vi "CMD_Loop.vi"() -> ()   [LabVIEW 2020, in "MotionMaster_SubCMD.lvlib"]
uses:
  MotionMaster_SubCMD.lvlib
  Cluster_CMD_CMD_Data.ctl
  ENUM_CMD_Mode.ctl
  ENUM_Pose List.ctl
  Shared Code/TypeDefs/Cluster_Pose Positions.ctl
  Shared Code/TypeDefs/Cluster_MotionMaster_Config Data.ctl
  Shared Code/TypeDefs/Cluster_Pose Name and  Data.ctl
  Lift/Cluster_CMD_ACT_Data.ctl
  Shared Code/TypeDefs/ENUM_Lift_CMD_Mode Select.ctl
  Wrist/Cluster_CMD_ACT_Data.ctl
  Shared Code/TypeDefs/ENUM_Wrist_CMD_Mode Select.ctl
  Extention/Cluster_CMD_ACT_Data.ctl
  Shared Code/TypeDefs/ENUM_Extend_CMD_Mode Select.ctl
  Shared Code/TypeDefs/Cluster_MotionMaster Output.ctl
  ENUM_CMD_State.ctl
  Shared Code/TypeDefs/Cluster_Lift_HW Outputs.ctl
  Shared Code/TypeDefs/Cluster_FX Sensor Values.ctl
  Shared Code/TypeDefs/Cluster_FX CloseLoop Values.ctl
  Shared Code/TypeDefs/Cluster_FX Limit Switchs.ctl
  Shared Code/TypeDefs/Cluster_FX Current Values.ctl
  Shared Code/TypeDefs/Cluster_FX Integrated Sensor Values.ctl
  Shared Code/TypeDefs/Cluster_Lift_SW Output Data.ctl
  Shared Code/TypeDefs/Cluster_Wrist HW Outputs.ctl
  Shared Code/TypeDefs/Cluster_Wrist_SW Output Data.ctl
  Shared Code/TypeDefs/Cluster_Extend HW Outputs.ctl
  Shared Code/TypeDefs/Cluster_Extend_SW Output Data.ctl
  ENUM_CMD_Action.ctl
  f0e3bde4-301b-4f9a-9fe5-06516af7aa09.vi
  30192d10-bba2-489c-a06e-f8bf0f82b926.vi
  77e6cb1f-e30f-4d03-9d33-3a90b036f1c5.vi
  37f9d8cc-f1a8-4678-af2d-79a500a222a4.vi
  5685669b-8200-4586-8aad-fb6ccbc2f0c7.vi
  9608b361-7489-41d5-b543-0e30ed415d4d.vi
  543e74ff-1c65-4f6d-a6cc-884adac36b74.vi
  2e6b047f-cb73-4edf-a9eb-2cc3cf528fa5.vi
  543e74ff-1c65-4f6d-a6cc-884adac36b74.vi/f38ca901-adc1-4ad8-996e-31aeb746ae36.vi
  543e74ff-1c65-4f6d-a6cc-884adac36b74.vi/958b2683-dd4b-41b7-8ed1-41c95f63cef0.vi
  2e6b047f-cb73-4edf-a9eb-2cc3cf528fa5.vi/f38ca901-adc1-4ad8-996e-31aeb746ae36.vi
  2e6b047f-cb73-4edf-a9eb-2cc3cf528fa5.vi/958b2683-dd4b-41b7-8ed1-41c95f63cef0.vi
  543e74ff-1c65-4f6d-a6cc-884adac36b74.vi/f38ca901-adc1-4ad8-996e-31aeb746ae36.vi/1c6bd52c-bbca-4d4a-a290-93ea2703fded.vi
  543e74ff-1c65-4f6d-a6cc-884adac36b74.vi/f38ca901-adc1-4ad8-996e-31aeb746ae36.vi/47c2b0d5-b5fa-444e-9535-611565d375db.vi
  2e6b047f-cb73-4edf-a9eb-2cc3cf528fa5.vi/f38ca901-adc1-4ad8-996e-31aeb746ae36.vi/1c6bd52c-bbca-4d4a-a290-93ea2703fded.vi
  2e6b047f-cb73-4edf-a9eb-2cc3cf528fa5.vi/f38ca901-adc1-4ad8-996e-31aeb746ae36.vi/47c2b0d5-b5fa-444e-9535-611565d375db.vi
  Global_CMD_CMD_Data In.vi
  Utility/Global_STOP.vi
  Lift/Global_ACT_Data Out.vi
  Wrist/Global_ACT_Data Out.vi
  Extention/Global_ACT_Data Out.vi
  <vilib>/Utility/Data Type/Get Type Information.vi
  <vilib>/Utility/error.llb/Trim Whitespace.vi
  Shared Code/Utility/RWA/RWA/File/RWA_PC FIle Read String.vi
  Shared Code/Utility/RWA/RWA/Read Write Anything/RWA_File String.vi
  Shared Code/Utility/RWA/RWA/File/RWA_PC File Write String.vi
  Global_CMD_Data Out.vi
  Lift/Global_CMD_ACT_Data In.vi
  Extention/Global_CMD_ACT_Data In.vi
  Wrist/Global_CMD_ACT_Data In.vi
  <vilib>/Comparison/Equal/Equal Functor/Equal Functor.lvclass
  Extention/Extend_ACT.lvlib
  Wrist/Wrist_ACT.lvlib
  Lift/Lift_ACT.lvlib
panel:
  out "Message":string
  out "Pose Index":i32
  out "Pose Targets":T1[](array[typedef])
  in  "Read Saved Config":bool
  in  "Update Config":bool
  out "MotionMaster_Output":T2
  out "Extend Position":i32
  out "Wrist @Positon":bool
  out "Wrist Position":i32
  out "Extend @ Positon":bool
  out "Lift Position":i32
  out "Lift @ Positon":bool
  out "Extend CMD":T4
  out "Wrist CMD":T6
  out "Lift CMD":T8
  out "CMD.ENABLE":bool
  out "Current Time":timestamp
  in  "Config Data":T10
  out "CMD":T12
  out "Cycle Time (S)":dbl format="%.3g"
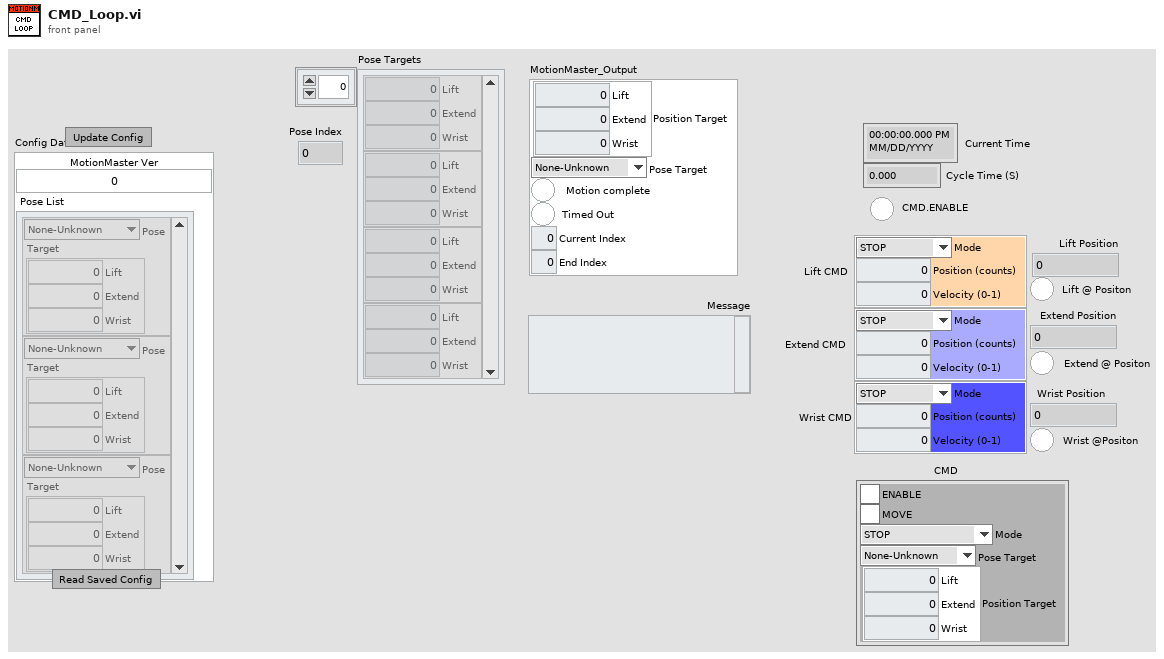
[diagram p1: front panel]
types:
  T1 = typedef "Cluster_Pose Positions.ctl" = cluster{"Lift":i32, "Extend":i32, "Wrist":i32}
  T2 = typedef "Cluster_MotionMaster Output.ctl" = cluster{"Position Target":T1, "Pose Target":T3, "Motion complete":bool, "Timed Out":bool, "Current Index":i32, "End Index":i32}
  T3 = typedef "MotionMaster_SubCMD.lvlib/ENUM_Pose List.ctl" = enum16{"None-Unknown", "Intake", "Score High", "Score Mid", "Safe Position", "Home Pos"}
  T4 = typedef "Extend_ACT.lvlib/Cluster_CMD_ACT_Data.ctl" = cluster{"Mode":T5, "Position (counts)":i32, "Velocity (0-1)":dbl}
  T5 = typedef "ENUM_Extend_CMD_Mode Select.ctl" = enum16{"STOP", "Position", "Velocity", "Force Home"}
  T6 = typedef "Wrist_ACT.lvlib/Cluster_CMD_ACT_Data.ctl" = cluster{"Mode":T7, "Position (counts)":i32, "Velocity (0-1)":dbl}
  T7 = typedef "ENUM_Wrist_CMD_Mode Select.ctl" = enum16{"STOP", "Position", "Speed"}
  T8 = typedef "Lift_ACT.lvlib/Cluster_CMD_ACT_Data.ctl" = cluster{"Mode":T9, "Position (counts)":i32, "Velocity (0-1)":dbl}
  T9 = typedef "ENUM_Lift_CMD_Mode Select.ctl" = enum16{"STOP", "Position", "Percent out"}
  T10 = typedef "Cluster_MotionMaster_Config Data.ctl" = cluster{"MotionMaster Ver":u64, "Pose List":T11[]}
  T11 = typedef "Cluster_Pose Name and  Data.ctl" = cluster{"Pose":T3, "Target":T1}
  T12 = typedef "MotionMaster_SubCMD.lvlib/Cluster_CMD_CMD_Data.ctl" = cluster{"ENABLE":bool, "MOVE":bool, "Mode":T13, "Pose Target":T3, "Position Target":T1}
  T13 = typedef "MotionMaster_SubCMD.lvlib/ENUM_CMD_Mode.ctl" = enum16{"STOP", "Pose Target", "Position Target"}
  T14 = typedef "Cluster_Extend_SW Output Data.ctl" = cluster{"Enabled":bool, "Closed Loop":bool, "exAt Positon":bool}
  T15 = typedef "Cluster_Extend HW Outputs.ctl" = cluster{"CLosed Loop":T16, "Limit Switches":T17, "Current":T18, "FX Encoder":T19, "Cancoder":T20}
  T16 = typedef "Cluster_FX CloseLoop Values.ctl" = cluster{"Target":dbl, "Error":i32, "Error D":dbl, "I Accum":dbl}
  T17 = typedef "Cluster_FX Limit Switchs.ctl" = cluster{"FWD Closed":bool, "REV Closed":bool}
  T18 = typedef "Cluster_FX Current Values.ctl" = cluster{"Supply":dbl, "Stator":dbl}
  T19 = typedef "Cluster_FX Sensor Values.ctl" = cluster{"Position":i32, "Velocity":i32}
  T20 = typedef "Cluster_FX Integrated Sensor Values.ctl" = cluster{"Position":dbl, "Velocity":dbl, "Absolute":dbl}
  T21 = typedef "Cluster_Wrist_SW Output Data.ctl" = cluster{"Enabled":bool, "Closed Loop":bool, "Wr At Positon":bool}
  T22 = typedef "Cluster_Wrist HW Outputs.ctl" = cluster{"Encoder":T19, "CLosed Loop":T16, "Limit Switches":T17, "Current":T18, "Cancoder":T20}
  T23 = typedef "Cluster_Lift_SW Output Data.ctl" = cluster{"Enabled":bool, "Closed Loop":bool, "At Positon":bool}
  T24 = typedef "Cluster_Lift_HW Outputs.ctl" = cluster{"Encoder":T19, "CLosed Loop":T16, "Limit Switches":T17, "Current":T18, "Cancoder":T20}
  T25 = typedef "MotionMaster_SubCMD.lvlib/ENUM_CMD_State.ctl" = enum16{"Startup", "Configuring", "Waining For Enable", "Waiting For Start", "Setting Pose", "Moving to Pose", "Shutdown", "Completing Pose"}
  T26 = cluster{"State":T25, "Previous State":T25, "Current Time":timestamp, "Previous Time":timestamp, "Start Time":timestamp, "Target Time (ms)":u32, "Cycle Time(S)":dbl, "CMD":T12, "Lift CMD":T8, "Extend CMD":T4, "Wrist CMD":T6, "Previous CMD":T12, "Lift HW":T24, "Lift SW":T23, "Wrist HW":T22, "Wrist SW":T21, "Extend HW":T15, "Extend SW":T14, "Config Data":T10, "ALL At Positon":bool, "Pose Index":i32, "Update Display":bool, "MotionMaster_Output":T2, "Team Files Folder":path, "Pose Array":T1[], "PoseName":T3, "Current Pose":T1, "Valid Pose Target":bool, "Pose Wait Time":dbl, "Message":string, "Max Move Time":dbl}
  T27 = enum16{"Done", "First Call", "First Check", "Enabled"}
  T28 = enum16{"Done", "First Call", "First Check", "Enabled", "Move Enabled", "Positions Not Set"}
  T29 = enum16{"Done", "First Call", "First Check", "Enabled", "Move Enabled", "Positions Set", "Not At Positon"}
  T30 = typedef "MotionMaster_SubCMD.lvlib/ENUM_CMD_Action.ctl" = enum16{"No Action", "Reset Time", "Reset All", "Set Pose", "Config Pose Read File", "Build Pose List", "Config SW File Read", "Config SW File Save", "Config From FP"}
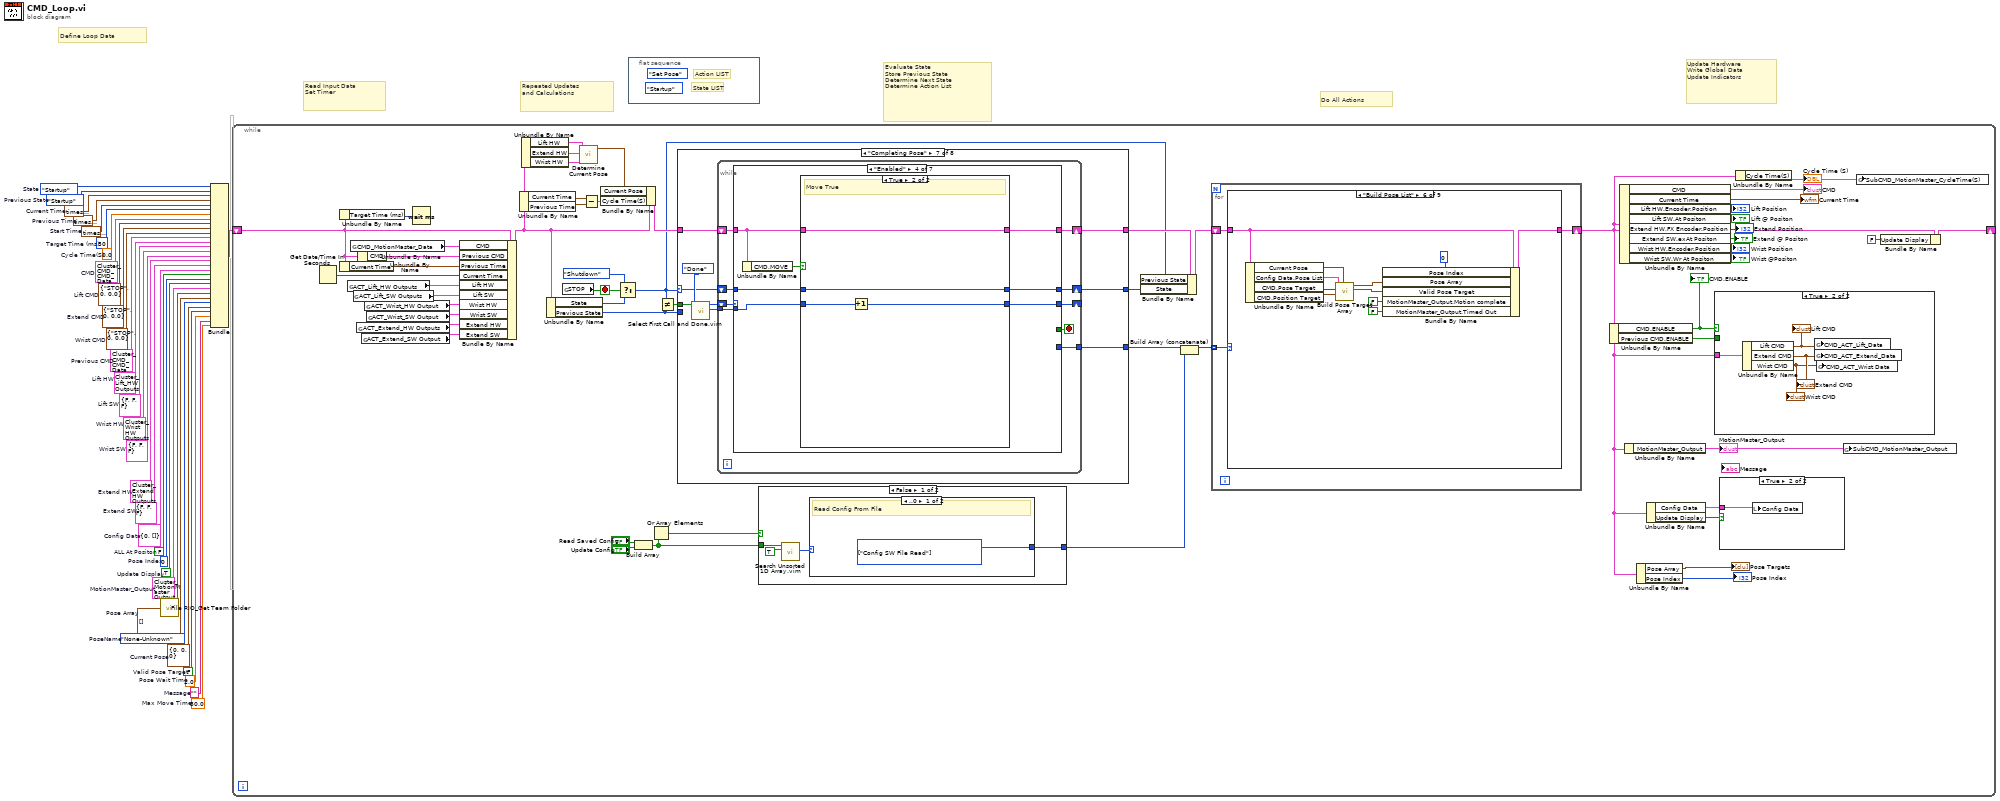
[diagram p0: block diagram]
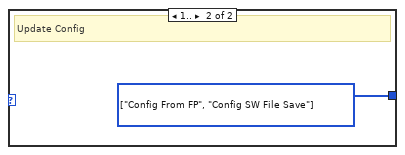
[diagram p2: hidden frame]
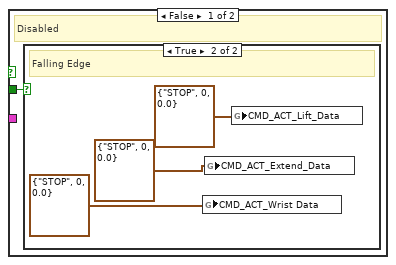
[diagram p5: hidden frame]
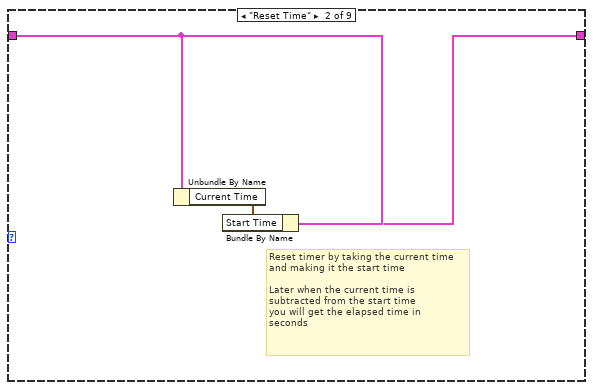
[diagram p8: hidden frame]
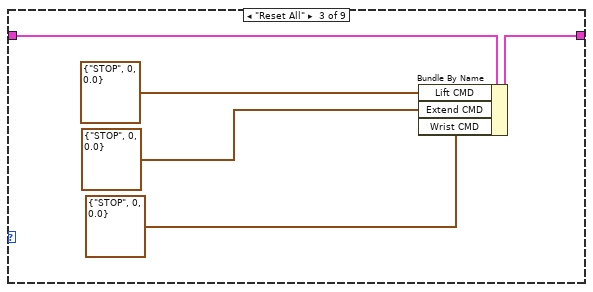
[diagram p9: hidden frame]
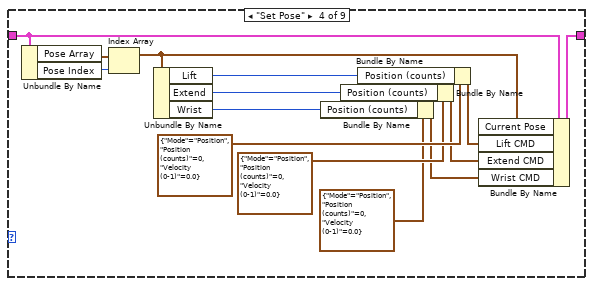
[diagram p10: hidden frame]
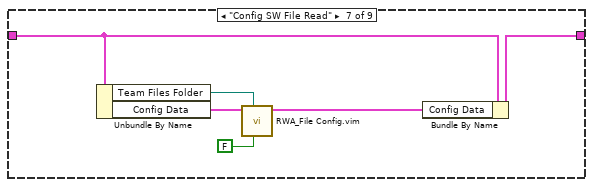
[diagram p12: hidden frame]
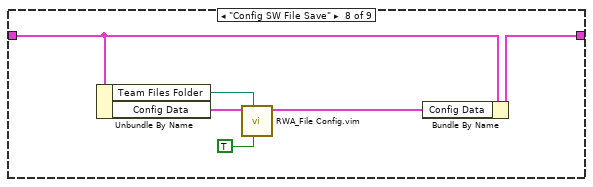
[diagram p13: hidden frame]
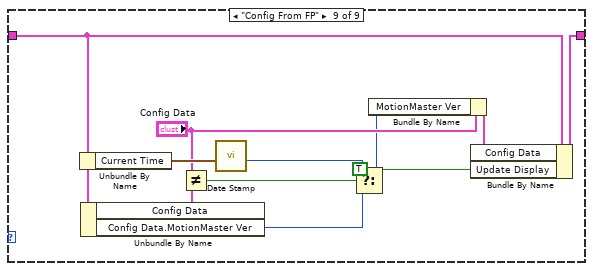
[diagram p14: hidden frame]
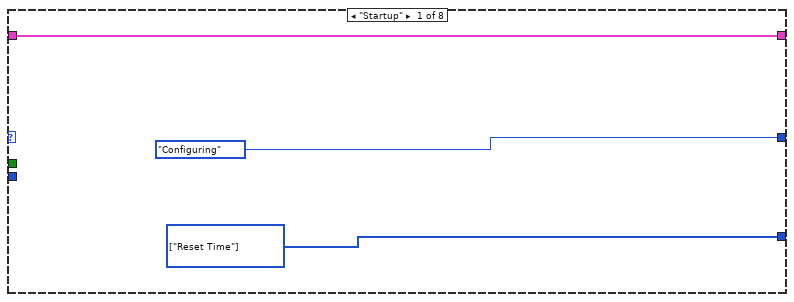
[diagram p15: hidden frame]
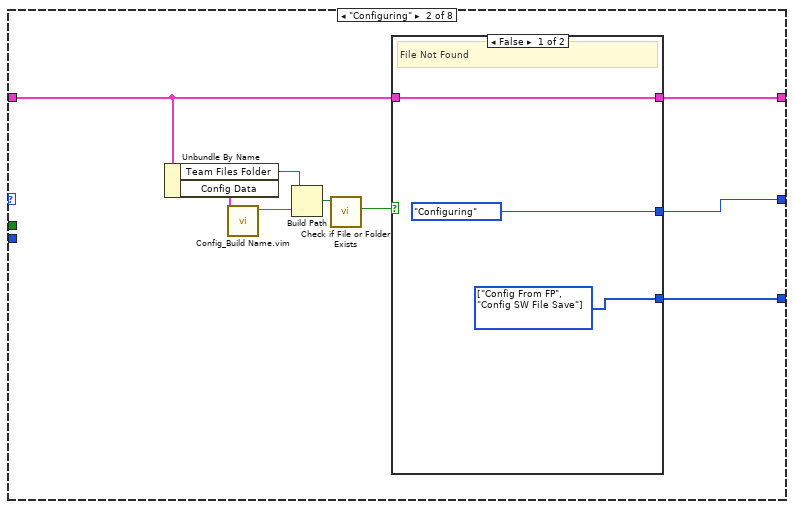
[diagram p16: hidden frame]
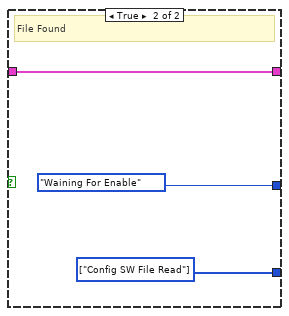
[diagram p17: hidden frame]
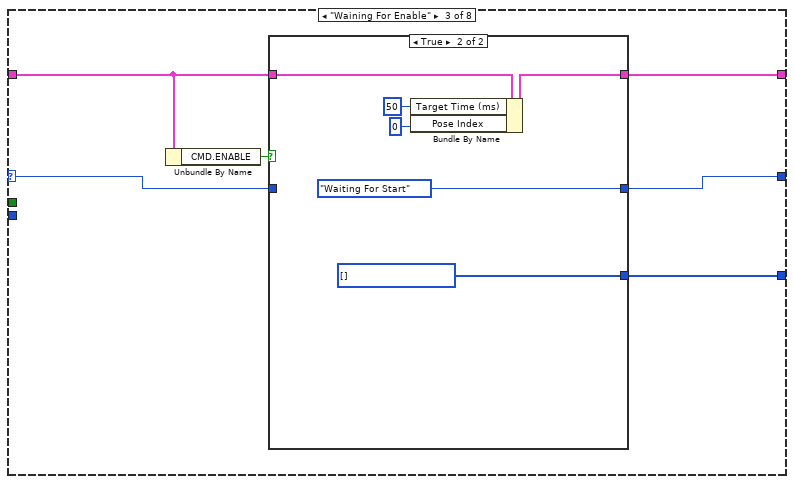
[diagram p18: hidden frame]
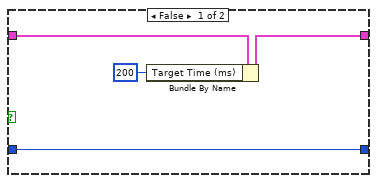
[diagram p19: hidden frame]
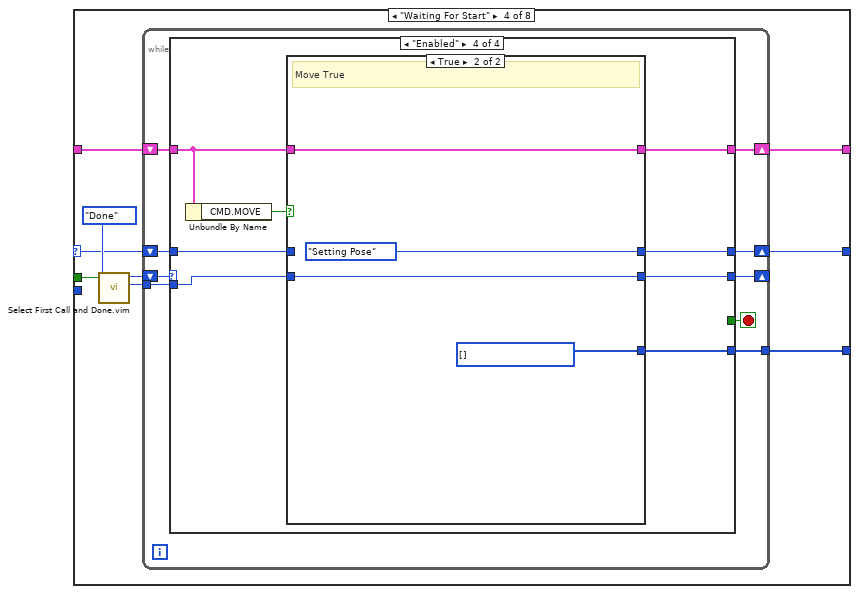
[diagram p20: hidden frame]
diagram:
  w1 = 30.0  # Max Move Time
  w2 = ""  # Message
  w3 = 2.0  # Pose Wait Time
  w4 = FALSE  # Valid Pose Target
  w5 = T1 {"Lift"=0, "Extend"=0, "Wrist"=0}  # Current Pose
  w6 = ENUM_Pose_List."None-Unknown"  # PoseName
  w8 = T1[] []  # Pose Array
  w10 = T2 {"Position Target"={"Lift"=0, "Extend"=0, "Wrist"=0}, "Pose Target"=enum."None-Unknown", "Motion complete"=FALSE, "Timed Out"=FALSE, "Current Index"=0, "End Index"=0}  # MotionMaster_Output
  w11 = TRUE  # Update Display
  w7 = 0  # Pose Index
  w12 = FALSE  # ALL At Positon
  w13 = T10 {"MotionMaster Ver"=0, "Pose List"=[]}  # Config Data
  w14 = T14 {"Enabled"=FALSE, "Closed Loop"=FALSE, "exAt Positon"=FALSE}  # Extend SW
  w15 = T15 {"CLosed Loop"={"Target"=0.0, "Error"=0, "Error D"=0.0, "I Accum"=0.0}, "Limit Switches"={"FWD Closed"=FALSE, "REV Closed"=FALSE}, "Current"={"Supply"=0.0, "Stator"=0.0}, "FX Encoder"={"Position"=0, "Velocity"=0}, "Cancoder"={"Position"=0.0, "Velocity"=0.0, "Absolute"=0.0}}  # Extend HW
  w16 = T21 {"Enabled"=FALSE, "Closed Loop"=FALSE, "Wr At Positon"=FALSE}  # Wrist SW
  w17 = T22 {"Encoder"={"Position"=0, "Velocity"=0}, "CLosed Loop"={"Target"=0.0, "Error"=0, "Error D"=0.0, "I Accum"=0.0}, "Limit Switches"={"FWD Closed"=FALSE, "REV Closed"=FALSE}, "Current"={"Supply"=0.0, "Stator"=0.0}, "Cancoder"={"Position"=0.0, "Velocity"=0.0, "Absolute"=0.0}}  # Wrist HW
  w18 = T23 {"Enabled"=FALSE, "Closed Loop"=FALSE, "At Positon"=FALSE}  # Lift SW
  w19 = T24 {"Encoder"={"Position"=0, "Velocity"=0}, "CLosed Loop"={"Target"=0.0, "Error"=0, "Error D"=0.0, "I Accum"=0.0}, "Limit Switches"={"FWD Closed"=FALSE, "REV Closed"=FALSE}, "Current"={"Supply"=0.0, "Stator"=0.0}, "Cancoder"={"Position"=0.0, "Velocity"=0.0, "Absolute"=0.0}}  # Lift HW
  w20 = T12 {"ENABLE"=FALSE, "MOVE"=FALSE, "Mode"=enum."STOP", "Pose Target"=enum."None-Unknown", "Position Target"={"Lift"=0, "Extend"=0, "Wrist"=0}}  # Previous CMD
  w21 = T6 {"Mode"=enum."STOP", "Position (counts)"=0, "Velocity (0-1)"=0.0}  # Wrist CMD
  w23 = T8 {"Mode"=enum."STOP", "Position (counts)"=0, "Velocity (0-1)"=0.0}  # Lift CMD
  w22 = T4 {"Mode"=enum."STOP", "Position (counts)"=0, "Velocity (0-1)"=0.0}  # Extend CMD
  w24 = 0.0  # Cycle Time(S)
  w25 = ENUM_CMD_State."Startup"  # Previous State
  w26 = timestamp(0 s since 1904-01-01)  # Previous Time
  w27 = u32 50  # Target Time (ms)
  w28 = T12 {"ENABLE"=FALSE, "MOVE"=FALSE, "Mode"=enum."STOP", "Pose Target"=enum."None-Unknown", "Position Target"={"Lift"=0, "Extend"=0, "Wrist"=0}}  # CMD
  w29 = timestamp(0 s since 1904-01-01)  # Start Time
  w30 = timestamp(0 s since 1904-01-01)  # Current Time
  w31 = ENUM_CMD_State."Startup"  # State
  # "Define Loop Data"
  # "Repeated Updates\nand Calculations"
  # "Read Input Data\nSet Timer"
  # "Evaluate State\nStore Previous State\nDetermine Next State\nDetermine Action List"
  # "Do All Actions"
  # "Update Hardware\nWrite Global Data\nUpdate Indicators"
  n1 = call "File RIO_Get Team Folder.vi"() -> ("Team Files Folder"=w9:path)  [unwired: 10 in, 1 out]
  n2 = Bundle("State"=w31, "Previous State"=w25, "Current Time"=w30, "Previous Time"=w26, "Start Time"=w29, "Target Time (ms)"=w27, "Cycle Time(S)"=w24, "CMD"=w28, "Lift CMD"=w23, "Extend CMD"=w22, "Wrist CMD"=w21, "Previous CMD"=w20, "Lift HW"=w19, "Lift SW"=w18, "Wrist HW"=w17, "Wrist SW"=w16, "Extend HW"=w15, "Extend SW"=w14, "Config Data"=w13, "ALL At Positon"=w12, "Pose Index"=w7, "Update Display"=w11, "MotionMaster_Output"=w10, "Team Files Folder"=w9, "Pose Array"=w8, "PoseName"=w6, "Current Pose"=w5, "Valid Pose Target"=w4, "Pose Wait Time"=w3, "Message"=w2, "Max Move Time"=w1) -> (w32:T26)  [unwired: 1 in]
  n3 = while {
    shift-right: [w46] -> _
    shift-left: w32 -> [w70]
    stop <- w76 stop-if-true
    n4 = Get Date/Time In Seconds() -> (seconds since 1Jan1904=w88:timestamp)
    n5 = Unbundle By Name(w70) -> ("Target Time (ms)"=w87:u32)
    n6 = Unbundle By Name(w70) -> ("Current Time"=w86:timestamp)
    n7 = global read "Global_ACT_Data Out.vi" "ACT_Lift_HW Outputs"() -> (w67:T24)
    n8 = global read "Global_CMD_CMD_Data In.vi" "CMD_MotionMaster_Data"() -> (w85:T12)
    n9 = global read "Global_ACT_Data Out.vi" "ACT_Lift_SW Outputs"() -> (w66:T23)
    n10 = global read "Global_ACT_Data Out.vi" "ACT_Extend_HW Outputs"() -> (w63:T15)
    n11 = Unbundle By Name(w70) -> ("CMD"=w69:T12)
    n12 = global read "Global_ACT_Data Out.vi" "ACT_Extend_SW Output"() -> (w62:T14)
    n13 = global read "Global_ACT_Data Out.vi" "ACT_Wrist_HW Output"() -> (w65:T22)
    n14 = global read "Global_ACT_Data Out.vi" "ACT_Wrist_SW Output"() -> (w64:T21)
    n15 = Wait (ms)(milliseconds to wait=w87) -> ()  [unwired: 1 out]
    n16 = Bundle By Name(cluster=w70, "CMD"=w85, "Previous CMD"=w69, "Previous Time"=w86, "Current Time"=w88, "Lift HW"=w67, "Lift SW"=w66, "Wrist HW"=w65, "Wrist SW"=w64, "Extend HW"=w63, "Extend SW"=w62) -> (w40:T26)
    n17 = Unbundle By Name(w40) -> ("Current Time"=w81:timestamp, "Previous Time"=w82:timestamp)
    n18 = Unbundle By Name(w40) -> ("Lift HW"=w39:T24, "Extend HW"=w38:T15, "Wrist HW"=w36:T22)
    n19 = Unbundle By Name(w40) -> ("State"=w83:T25, "Previous State"=w35:T25)
    n20 = global read "Global_STOP.vi" "STOP"() -> (w76:bool)
    n21 = call "Determine Current Pose.vi"("Wrist HW"=w36, "Extend HW"=w38, "Lift HW"=w39) -> ("Current Pose Out"=w37:T1)  [unwired: 8 in]
    n22 = Subtract(x=w81, y=w82) -> (x-y=w80:dbl)
    n23 = Bundle By Name(cluster=w40, "Current Pose"=w37, "Cycle Time(S)"=w80) -> (w77:T26)
    n24 = Select(t=ENUM_CMD_State."Shutdown" ("State"), s=w76, f=w83) -> (s? t:f=w34:T25)
    n25 = Build Array("Read Saved Config", "Update Config") -> (w48:bool[])
    n26 = Or Array Elements(Boolean array=w48) -> (logical OR=w49:bool)
    n27 = Not Equal?(x=w34, y=w35) -> (x != y?=w33:bool)
    n28 = case shown="\"Completing Pose\"" w34 {
      selector: w34 -> [_ _ w185 w199 w255 w354 w476 _]
      tunnel: w77 -> [w167 w171 w187 w207 w263 w362 w484 w610]
      tunnel: [w167 w170 w186 w206 w262 w361 w483 w610] -> w74
      tunnel: [ENUM_CMD_State."Configuring" ("State") w168 w184 w205 w261 w360 w482 ENUM_CMD_State."Shutdown" ("State")] -> w73
      tunnel: [w166 w169 w183 w204 w260 w359 w481 w608] -> w72
      tunnel: w35 -> [_ _ _ _ _ _ _ _]
      tunnel: w33 -> [_ _ _ w203 w259 w358 w480 _]
      frame "Startup" {
        w166 = T30[] [enum."Reset Time"] items=["No Action", "Reset Time", "Reset All", "Set Pose", "Config Pose Read File", "Build Pose List", "Config SW File Read", "Config SW File Save", "Config From FP"] ("Actions")
      }
      frame "Configuring" {
        n29 = Unbundle By Name(w171) -> ("Team Files Folder"=w173:path, "Config Data"=w174:T10)
        n30 = call "Config_Build Name.vim"("Config First Name"=w174) -> ("Cfg file"=w176:string)  [unwired: 9 in, 1 out]
        n31 = Build Path(base path=w173, name or relative path=w176) -> (appended path=w175:path)
        n32 = call <vilib>:"Check if File or Folder Exists.vi"("path"=w175) -> ("file or folder exists?"=w172:bool)  [unwired: 8 in, 2 out]
        n33 = case shown="False" w172 {
          tunnel: w171 -> [w179 w182]
          tunnel: [w179 w182] -> w170
          tunnel: [w177 w181] -> w169
          tunnel: [ENUM_CMD_State."Configuring" ("State") ENUM_CMD_State."Waining For Enable" ("State")] -> w168
          frame False {
            w177 = T30[] [enum."Config From FP", enum."Config SW File Save"] items=["No Action", "Reset Time", "Reset All", "Set Pose", "Config Pose Read File", "Build Pose List", "Config SW File Read", "Config SW File Save", "Config From FP"] ("appended array")
            # "File Not Found"
          }
          frame True {
            w181 = T30[] [enum."Config SW File Read"] items=["No Action", "Reset Time", "Reset All", "Set Pose", "Config Pose Read File", "Build Pose List", "Config SW File Read", "Config SW File Save", "Config From FP"] ("appended array")
            # "File Found"
          }
        }
      }
      frame "Waining For Enable" {
        n34 = Unbundle By Name(w187) -> ("CMD.ENABLE"=w188:bool)
        n35 = case shown="True" w188 {
          tunnel: w187 -> [w191 w197]
          tunnel: [w192 w198] -> w186
          tunnel: w185 -> [w189 _]
          tunnel: [w189 ENUM_CMD_State."Waiting For Start" ("State")] -> w184
          tunnel: [_ w194] -> w183
          frame False {
            n36 = Bundle By Name(cluster=w191, "Target Time (ms)"=u32 200) -> (w192:T26)
          }
          frame True {
            w194 = T30[] [] items=["No Action", "Reset Time", "Reset All", "Set Pose", "Config Pose Read File", "Build Pose List", "Config SW File Read", "Config SW File Save", "Config From FP"] ("Actions")
            n37 = Bundle By Name(cluster=w197, "Target Time (ms)"=u32 50, "Pose Index"=0) -> (w198:T26)
          }
        }
      }
      frame "Waiting For Start" {
        n38 = call "Select First Call and Done.vim"("First Call"=w203, "Enum 3"=T27."Done") -> ("DONE Select"=w201:T27, "First Call Select"=w202:T27)  [unwired: 8 in]
        n39 = while {
          tunnel: [w213] -> w204
          shift-right: [w215] -> w206
          shift-left: w207 -> [w216]
          shift-right: [w211] -> _
          shift-left: w202 -> [w212]
          tunnel: w201 -> [w210]
          shift-right: [w214] -> w205
          shift-left: w199 -> [w208]
          stop <- w209 stop-if-true
          n40 = case shown="\"Enabled\"" w212 {
            selector: w212 -> [_ w223 w226 _]
            tunnel: w216 -> [w218 w221 w231 w246]
            tunnel: [w218 w221 w230 w245] -> w215
            tunnel: [w217 w224 w229 w244] -> w214
            tunnel: [_ _ _ w240] -> w213
            tunnel: [w220 w222 w228 w243] -> w211
            tunnel: w210 -> [w220 _ w225 w242]
            tunnel: [TRUE _ _ _] -> w209
            tunnel: w208 -> [w217 w224 w227 w241]
            frame "Done" {
            }
            frame "First Call" {
              n41 = Increment(x=w223) -> (x+1=w222:T27)
            }
            frame "First Check" {
              n42 = Unbundle By Name(w231) -> ("CMD.ENABLE"=w232:bool)
              n43 = case shown="False" w232 {
                tunnel: w231 -> [w235 w238]
                tunnel: [w235 w238] -> w230
                tunnel: [ENUM_CMD_State."Waining For Enable" ("State") w237] -> w229
                tunnel: [w233 w236] -> w228
                tunnel: w226 -> [_ w239]
                tunnel: w227 -> [_ w237]
                tunnel: w225 -> [w233 _]
                frame False {
                  # "Disabled"
                }
                frame True {
                  # "Enable True"
                  n44 = Increment(x=w239) -> (x+1=w236:T27)
                }
              }
            }
            frame "Enabled" {
              n45 = Unbundle By Name(w246) -> ("CMD.MOVE"=w247:bool)
              n46 = case shown="True" w247 {
                tunnel: w246 -> [w250 w254]
                tunnel: [w250 w254] -> w245
                tunnel: [ENUM_CMD_State."Waiting For Start" ("State") ENUM_CMD_State."Setting Pose" ("State")] -> w244
                tunnel: [w248 w253] -> w243
                tunnel: w242 -> [w248 w253]
                tunnel: w241 -> [_ _]
                tunnel: [_ w251] -> w240
                frame False {
                  # "Disabled"
                }
                frame True {
                  w251 = T30[] [] items=["No Action", "Reset Time", "Reset All", "Set Pose", "Config Pose Read File", "Build Pose List", "Config SW File Read", "Config SW File Save", "Config From FP"] ("Actions")
                  # "Move True"
                }
              }
            }
          }
        }
      }
      frame "Setting Pose" {
        n47 = call "Select First Call and Done.vim"("First Call"=w259, "Enum 3"=T28."Done" ("Enum")) -> ("DONE Select"=w257:T28, "First Call Select"=w258:T28)  [unwired: 8 in]
        n48 = while {
          tunnel: [w269] -> w260
          shift-right: [w271] -> w262
          shift-left: w263 -> [w272]
          shift-right: [w267] -> _
          shift-left: w258 -> [w268]
          tunnel: w257 -> [w266]
          shift-right: [w270] -> w261
          shift-left: w255 -> [w264]
          stop <- w265 stop-if-true
          n49 = case shown="\"Enabled\"" w268 {
            selector: w268 -> [_ _ w284 _ w313 w340]
            tunnel: w272 -> [w274 w278 w289 w303 w322 w341]
            tunnel: [w274 w279 w288 w302 w328 w347] -> w271
            tunnel: [w273 w282 w287 w301 w327 w346] -> w270
            tunnel: [_ w280 _ _ _ _] -> w269
            tunnel: [w276 w281 w286 w300 w326 w345] -> w267
            tunnel: w266 -> [w276 w281 w283 w299 w312 w339]
            tunnel: [TRUE _ _ _ _ _] -> w265
            tunnel: w264 -> [w273 w282 w285 w298 w325 w344]
            frame "Done" {
            }
            frame "First Call" {
              w280 = T30[] [enum."Build Pose List", enum."Set Pose"] items=["No Action", "Reset Time", "Reset All", "Set Pose", "Config Pose Read File", "Build Pose List", "Config SW File Read", "Config SW File Save", "Config From FP"] ("Actions")
              n50 = Unbundle By Name(w278) -> ("Current Time"=w277:timestamp)
              n51 = Bundle By Name(cluster=w278, "Start Time"=w277) -> (w279:T26)
            }
            frame "First Check" {
              n52 = Unbundle By Name(w289) -> ("CMD.ENABLE"=w290:bool)
              n53 = case shown="True" w290 {
                tunnel: w289 -> [w293 w296]
                tunnel: [w293 w296] -> w288
                tunnel: [ENUM_CMD_State."Waining For Enable" ("State") w295] -> w287
                tunnel: [w291 w294] -> w286
                tunnel: w284 -> [_ w297]
                tunnel: w285 -> [_ w295]
                tunnel: w283 -> [w291 _]
                frame False {
                  # "Disabled"
                }
                frame True {
                  # "Enable True"
                  n54 = Increment(x=w297) -> (x+1=w294:T28)
                }
              }
            }
            frame "Enabled" {
              n55 = Unbundle By Name(w303) -> ("CMD.MOVE"=w304:bool)
              n56 = case shown="True" w304 {
                tunnel: w303 -> [w307 w311]
                tunnel: [w307 w311] -> w302
                tunnel: [ENUM_CMD_State."Waiting For Start" ("State") w309] -> w301
                tunnel: [w305 w308] -> w300
                tunnel: w299 -> [w305 w310]
                tunnel: w298 -> [_ w309]
                frame False {
                  # "Disabled"
                }
                frame True {
                  # "Move True"
                  n57 = Increment(x=w310) -> (x+1=w308:T28)
                }
              }
            }
            frame "Move Enabled" {
              n58 = Unbundle By Name(w322) -> ("Extend HW.FX Encoder.Position"=w321:i32, "Current Pose.Extend"=w320:i32)
              n59 = Unbundle By Name(w322) -> ("Wrist HW.Encoder.Position"=w319:i32, "Current Pose.Wrist"=w318:i32)
              n60 = Unbundle By Name(w322) -> ("Lift HW.Encoder.Position"=w324:i32, "Current Pose.Lift"=w323:i32)
              n61 = Equal?(x=w324, y=w323) -> (x = y?=w316:bool)
              n62 = Equal?(x=w319, y=w318) -> (x = y?=w315:bool)
              n63 = Equal?(x=w321, y=w320) -> (x = y?=w317:bool)
              n64 = Compound Arithmetic op=AND(w316, w317, w315) -> (w314:bool)
              n65 = case shown="True" w314 {
                tunnel: w322 -> [w332 w335]
                tunnel: [w332 w335] -> w328
                tunnel: [w330 ENUM_CMD_State."Moving to Pose" ("State")] -> w327
                tunnel: [w329 w334] -> w326
                tunnel: w313 -> [w331 _]
                tunnel: w325 -> [w330 _]
                tunnel: w312 -> [_ w334]
                frame False {
                  # "Positions Not Set"
                  n66 = Increment(x=w331) -> (x+1=w329:T28)
                }
                frame True {
                  # "Positions Set"
                }
              }
            }
            frame "Positions Not Set" {
              n67 = Unbundle By Name(w341) -> ("Current Time"=w343:timestamp, "Start Time"=w342:timestamp, "Pose Wait Time"=w338:dbl)
              n68 = Subtract(x=w343, y=w342) -> (x-y=w337:dbl)
              n69 = Greater Or Equal?(x=w337, y=w338) -> (x >= y?=w336:bool)
              n70 = case shown="True" w336 {
                tunnel: w341 -> [w350 w353]
                tunnel: [w350 w353] -> w347
                tunnel: [w349 ENUM_CMD_State."Waiting For Start" ("State")] -> w346
                tunnel: [w348 w352] -> w345
                tunnel: w340 -> [_ _]
                tunnel: w344 -> [w349 _]
                tunnel: w339 -> [w348 w352]
                frame False {
                  # "Time Not Expired"
                }
                frame True {
                  # "Time Expired"
                }
              }
            }
          }
        }
      }
      frame "Moving to Pose" {
        n71 = call "Select First Call and Done.vim"("First Call"=w358, "Enum 3"=T29."Done" ("Enum")) -> ("DONE Select"=w356:T29, "First Call Select"=w357:T29)  [unwired: 8 in]
        n72 = while {
          tunnel: [w368] -> w359
          shift-right: [w370] -> w361
          shift-left: w362 -> [w371]
          shift-right: [w366] -> _
          shift-left: w357 -> [w367]
          tunnel: w356 -> [w365]
          shift-right: [w369] -> w360
          shift-left: w354 -> [w363]
          stop <- w364 stop-if-true
          n73 = case shown="\"Enabled\"" w367 {
            selector: w367 -> [_ w378 w384 _ w413 w441 w460]
            tunnel: w371 -> [w373 w380 w389 w403 w422 w442 w461]
            tunnel: [w373 w381 w388 w402 w428 w446 w465] -> w370
            tunnel: [w372 w382 w387 w401 w427 w445 w464] -> w369
            tunnel: [_ w376 _ _ _ _ _] -> w368
            tunnel: [w375 w377 w386 w400 w426 w444 w463] -> w366
            tunnel: w365 -> [w375 _ w383 w399 w412 w440 w459]
            tunnel: [TRUE _ _ _ _ _ _] -> w364
            tunnel: w363 -> [w372 w382 w385 w398 w425 w443 w462]
            frame "Done" {
            }
            frame "First Call" {
              w376 = T30[] [] items=["No Action", "Reset Time", "Reset All", "Set Pose", "Config Pose Read File", "Build Pose List", "Config SW File Read", "Config SW File Save", "Config From FP"] ("Actions")
              n74 = Increment(x=w378) -> (x+1=w377:T29)
              n75 = Unbundle By Name(w380) -> ("Current Time"=w379:timestamp)
              n76 = Bundle By Name(cluster=w380, "Start Time"=w379) -> (w381:T26)
            }
            frame "First Check" {
              n77 = Unbundle By Name(w389) -> ("CMD.ENABLE"=w390:bool)
              n78 = case shown="True" w390 {
                tunnel: w389 -> [w393 w396]
                tunnel: [w393 w396] -> w388
                tunnel: [ENUM_CMD_State."Waining For Enable" ("State") w395] -> w387
                tunnel: [w391 w394] -> w386
                tunnel: w384 -> [_ w397]
                tunnel: w385 -> [_ w395]
                tunnel: w383 -> [w391 _]
                frame False {
                  # "Disabled"
                }
                frame True {
                  # "Enable True"
                  n79 = Increment(x=w397) -> (x+1=w394:T29)
                }
              }
            }
            frame "Enabled" {
              n80 = Unbundle By Name(w403) -> ("CMD.MOVE"=w404:bool)
              n81 = case shown="True" w404 {
                tunnel: w403 -> [w407 w411]
                tunnel: [w407 w411] -> w402
                tunnel: [ENUM_CMD_State."Waiting For Start" ("State") w409] -> w401
                tunnel: [w405 w408] -> w400
                tunnel: w399 -> [w405 w410]
                tunnel: w398 -> [_ w409]
                frame False {
                  # "Disabled"
                }
                frame True {
                  # "Move True"
                  n82 = Increment(x=w410) -> (x+1=w408:T29)
                }
              }
            }
            frame "Move Enabled" {
              n83 = Unbundle By Name(w422) -> ("Extend HW.FX Encoder.Position"=w421:i32, "Current Pose.Extend"=w420:i32)
              n84 = Unbundle By Name(w422) -> ("Wrist HW.Encoder.Position"=w419:i32, "Current Pose.Wrist"=w418:i32)
              n85 = Unbundle By Name(w422) -> ("Lift HW.Encoder.Position"=w424:i32, "Current Pose.Lift"=w423:i32)
              n86 = Equal?(x=w424, y=w423) -> (x = y?=w416:bool)
              n87 = Equal?(x=w419, y=w418) -> (x = y?=w415:bool)
              n88 = Equal?(x=w421, y=w420) -> (x = y?=w417:bool)
              n89 = Compound Arithmetic op=AND(w416, w417, w415) -> (w414:bool)
              n90 = case shown="True" w414 {
                tunnel: w422 -> [w431 w435]
                tunnel: [w431 w435] -> w428
                tunnel: [ENUM_CMD_State."Setting Pose" ("State") w432] -> w427
                tunnel: [w430 w433] -> w426
                tunnel: w413 -> [_ w434]
                tunnel: w425 -> [_ w432]
                tunnel: w412 -> [w430 _]
                frame False {
                  # "Positions Not Set"
                }
                frame True {
                  # "Positions Set"
                  n91 = Increment(x=w434) -> (x+1=w433:T29)
                }
              }
            }
            frame "Positions Set" {
              n92 = Unbundle By Name(w442) -> ("Lift SW.At Positon"=w438:bool, "Extend SW.exAt Positon"=w439:bool, "Wrist SW.Wr At Positon"=w437:bool)
              n93 = Compound Arithmetic op=AND(w438, w439, w437) -> (w436:bool)
              n94 = case shown="False" w436 {
                tunnel: w442 -> [w450 w453]
                tunnel: [w450 w453] -> w446
                tunnel: [w449 ENUM_CMD_State."Completing Pose" ("State")] -> w445
                tunnel: [w447 w452] -> w444
                tunnel: w441 -> [w448 _]
                tunnel: w443 -> [w449 _]
                tunnel: w440 -> [_ w452]
                frame False {
                  # "Not At Pose"
                  n95 = Increment(x=w448) -> (x+1=w447:T29)
                }
                frame True {
                  # "Pose Complete"
                }
              }
            }
            frame "Not At Positon" {
              n96 = Unbundle By Name(w461) -> ("Current Time"=w458:timestamp, "Start Time"=w457:timestamp, "Pose Wait Time"=w455:dbl)
              n97 = Subtract(x=w458, y=w457) -> (x-y=w456:dbl)
              n98 = Greater Or Equal?(x=w456, y=w455) -> (x >= y?=w454:bool)
              n99 = case shown="False" w454 {
                tunnel: w461 -> [w466 w472]
                tunnel: [w467 w473] -> w465
                tunnel: [ENUM_CMD_State."Moving to Pose" ("State") ENUM_CMD_State."Moving to Pose" ("State")] -> w464
                tunnel: [w470 w475] -> w463
                tunnel: w460 -> [_ _]
                tunnel: w462 -> [_ _]
                tunnel: w459 -> [w470 w475]
                frame False {
                  # "Time Not Expired"
                  n100 = Bundle By Name(cluster=w466, "Message"="Moving to Pose") -> (w467:T26)
                }
                frame True {
                  # "Time Expired"
                  n101 = Bundle By Name(cluster=w472, "Message"="MOVE Time Expired") -> (w473:T26)
                }
              }
            }
          }
        }
      }
      frame "Completing Pose" {
        n102 = call "Select First Call and Done.vim"("First Call"=w480, "Enum 3"=T29."Done" ("Enum")) -> ("DONE Select"=w478:T29, "First Call Select"=w479:T29)  [unwired: 8 in]
        n103 = while {
          tunnel: [w490] -> w481
          shift-right: [w492] -> w483
          shift-left: w484 -> [w493]
          shift-right: [w488] -> _
          shift-left: w479 -> [w489]
          tunnel: w478 -> [w487]
          shift-right: [w491] -> w482
          shift-left: w476 -> [w485]
          stop <- w486 stop-if-true
          n104 = case shown="\"Enabled\"" w489 {
            selector: w489 -> [_ w500 w511 _ w545 w573 w592]
            tunnel: w493 -> [w495 w502 w516 w535 w554 w574 w593]
            tunnel: [w495 w503 w515 w534 w560 w578 w597] -> w492
            tunnel: [w494 w504 w514 w533 w559 w577 w596] -> w491
            tunnel: [_ w498 _ _ _ _ _] -> w490
            tunnel: [w497 w499 w513 w532 w558 w576 w595] -> w488
            tunnel: w487 -> [w497 _ w510 w531 w544 w572 w591]
            tunnel: [TRUE _ _ _ _ _ _] -> w486
            tunnel: w485 -> [w494 w504 w512 w530 w557 w575 w594]
            frame "Done" {
            }
            frame "First Call" {
              w498 = T30[] [] items=["No Action", "Reset Time", "Reset All", "Set Pose", "Config Pose Read File", "Build Pose List", "Config SW File Read", "Config SW File Save", "Config From FP"] ("Actions")
              n105 = Increment(x=w500) -> (x+1=w499:T29)
              n106 = Unbundle By Name(w502) -> ("Current Time"=w501:timestamp)
              n107 = Bundle By Name(cluster=w502, "Start Time"=w501) -> (w503:T26)
            }
            frame "First Check" {
              n108 = Unbundle By Name(w516) -> ("Pose Index"=w505:i32, "Pose Array"=w509:T1[])
              n109 = Array Size(array=w509) -> (size(s)=w508:i32)
              n110 = Decrement(x=w508) -> (x-1=w507:i32)
              n111 = Greater Or Equal?(x=w505, y=w507) -> (x >= y?=w506:bool)
              n112 = case shown="True" w506 {
                tunnel: w516 -> [w518 w526]
                tunnel: [w519 w527] -> w515
                tunnel: [ENUM_CMD_State."Setting Pose" ("State") w529] -> w514
                tunnel: [w521 w528] -> w513
                tunnel: w511 -> [_ _]
                tunnel: w512 -> [_ w529]
                tunnel: w510 -> [w521 w528]
                tunnel: w505 -> [w520 _]
                frame False {
                  # "Continue to next pose"
                  n113 = Increment(x=w520) -> (x+1=w517:i32)
                  n114 = Bundle By Name(cluster=w518, "Pose Index"=w517) -> (w519:T26)
                }
                frame True {
                  # "Last Pose Complete"
                  n115 = Bundle By Name(cluster=w526, "MotionMaster_Output.Timed Out"=FALSE, "MotionMaster_Output.Motion complete"=TRUE, "Message"="POSE Complete") -> (w527:T26)
                }
              }
            }
            frame "Enabled" {
              n116 = Unbundle By Name(w535) -> ("CMD.MOVE"=w536:bool)
              n117 = case shown="True" w536 {
                tunnel: w535 -> [w539 w543]
                tunnel: [w539 w543] -> w534
                tunnel: [ENUM_CMD_State."Waiting For Start" ("State") w541] -> w533
                tunnel: [w537 w540] -> w532
                tunnel: w531 -> [w537 w542]
                tunnel: w530 -> [_ w541]
                frame False {
                  # "Disabled"
                }
                frame True {
                  # "Move True"
                  n118 = Increment(x=w542) -> (x+1=w540:T29)
                }
              }
            }
            frame "Move Enabled" {
              n119 = Unbundle By Name(w554) -> ("Extend HW.FX Encoder.Position"=w553:i32, "Current Pose.Extend"=w552:i32)
              n120 = Unbundle By Name(w554) -> ("Wrist HW.Encoder.Position"=w551:i32, "Current Pose.Wrist"=w550:i32)
              n121 = Unbundle By Name(w554) -> ("Lift HW.Encoder.Position"=w556:i32, "Current Pose.Lift"=w555:i32)
              n122 = Equal?(x=w556, y=w555) -> (x = y?=w548:bool)
              n123 = Equal?(x=w551, y=w550) -> (x = y?=w547:bool)
              n124 = Equal?(x=w553, y=w552) -> (x = y?=w549:bool)
              n125 = Compound Arithmetic op=AND(w548, w549, w547) -> (w546:bool)
              n126 = case shown="True" w546 {
                tunnel: w554 -> [w563 w567]
                tunnel: [w563 w567] -> w560
                tunnel: [ENUM_CMD_State."Setting Pose" ("State") w564] -> w559
                tunnel: [w562 w565] -> w558
                tunnel: w545 -> [_ w566]
                tunnel: w557 -> [_ w564]
                tunnel: w544 -> [w562 _]
                frame False {
                  # "Positions Not Set"
                }
                frame True {
                  # "Positions Set"
                  n127 = Increment(x=w566) -> (x+1=w565:T29)
                }
              }
            }
            frame "Positions Set" {
              n128 = Unbundle By Name(w574) -> ("Lift SW.At Positon"=w570:bool, "Extend SW.exAt Positon"=w571:bool, "Wrist SW.Wr At Positon"=w569:bool)
              n129 = Compound Arithmetic op=AND(w570, w571, w569) -> (w568:bool)
              n130 = case shown="False" w568 {
                tunnel: w574 -> [w582 w585]
                tunnel: [w582 w585] -> w578
                tunnel: [w581 ENUM_CMD_State."Completing Pose" ("State")] -> w577
                tunnel: [w579 w584] -> w576
                tunnel: w573 -> [w580 _]
                tunnel: w575 -> [w581 _]
                tunnel: w572 -> [_ w584]
                frame False {
                  # "Not At Pose"
                  n131 = Increment(x=w580) -> (x+1=w579:T29)
                }
                frame True {
                  # "Pose Complete"
                }
              }
            }
            frame "Not At Positon" {
              n132 = Unbundle By Name(w593) -> ("Current Time"=w590:timestamp, "Start Time"=w589:timestamp, "Pose Wait Time"=w587:dbl)
              n133 = Subtract(x=w590, y=w589) -> (x-y=w588:dbl)
              n134 = Greater Or Equal?(x=w588, y=w587) -> (x >= y?=w586:bool)
              n135 = case shown="False" w586 {
                tunnel: w593 -> [w598 w604]
                tunnel: [w599 w605] -> w597
                tunnel: [ENUM_CMD_State."Moving to Pose" ("State") ENUM_CMD_State."Moving to Pose" ("State")] -> w596
                tunnel: [w602 w607] -> w595
                tunnel: w592 -> [_ _]
                tunnel: w594 -> [_ _]
                tunnel: w591 -> [w602 w607]
                frame False {
                  # "Time Not Expired"
                  n136 = Bundle By Name(cluster=w598, "Message"="Moving to Pose") -> (w599:T26)
                }
                frame True {
                  # "Time Expired"
                  n137 = Bundle By Name(cluster=w604, "Message"="MOVE Time Expired") -> (w605:T26)
                }
              }
            }
          }
        }
      }
      frame "Shutdown" {
        w608 = T30[] [enum."Reset All"] items=["No Action", "Reset Time", "Reset All", "Set Pose", "Config Pose Read File", "Build Pose List", "Config SW File Read", "Config SW File Save", "Config From FP"] ("Actions")
      }
    }
    n138 = case shown="False" w49 {
      tunnel: w48 -> [w91 _]
      tunnel: [w89 _] -> w47
      frame False {
        n139 = call "Search Unsorted 1D Array.vim"("element"=TRUE, "unsorted 1D array"=w91) -> ("index of element"=w90:i32)  [unwired: 9 in]
        n140 = case shown="..0" w90 {
          tunnel: [w93 w94] -> w89
          frame ..0 {
            w93 = T30[] [enum."Config SW File Read"] items=["No Action", "Reset Time", "Reset All", "Set Pose", "Config Pose Read File", "Build Pose List", "Config SW File Read", "Config SW File Save", "Config From FP"] ("array")
            # "Read Config From File"
          }
          frame 1.. {
            w94 = T30[] [enum."Config From FP", enum."Config SW File Save"] items=["No Action", "Reset Time", "Reset All", "Set Pose", "Config Pose Read File", "Build Pose List", "Config SW File Read", "Config SW File Save", "Config From FP"] ("array")
            # "Update Config"
          }
        }
      }
      frame True {
      }
    }
    n141 = Bundle By Name(cluster=w74, "Previous State"=w34, "State"=w73) -> (w75:T26)
    n142 = Build Array (concatenate)(w72, w47) -> (w52:T30[])
    n143 = for {
      tunnel: w52 -> [w106] mode=indexing
      shift-right: [w105] -> w43
      shift-left: w75 -> [w104]
      n144 = case shown="\"Build Pose List\"" w106 {
        tunnel: w104 -> [w107 w110 w114 w126 w130 w139 w146 w152 w162]
        tunnel: [w107 w109 w115 w127 w130 w140 w147 w153 w164] -> w105
        frame "No Action" {
        }
        frame "Reset Time" {
          # "Reset timer by taking the current time\nand making it the start time\n\nLater when the current time is \nsubtracted from the start time\nyou will get the elapsed time in \nseconds"
          n145 = Unbundle By Name(w110) -> ("Current Time"=w108:timestamp)
          n146 = Bundle By Name(cluster=w110, "Start Time"=w108) -> (w109:T26)
        }
        frame "Reset All" {
          n147 = Bundle By Name(cluster=w114, "Lift CMD"=T8 {"Mode"=enum."STOP", "Position (counts)"=0, "Velocity (0-1)"=0.0} ("Sholder CMD"), "Extend CMD"=T4 {"Mode"=enum."STOP", "Position (counts)"=0, "Velocity (0-1)"=0.0}, "Wrist CMD"=T6 {"Mode"=enum."STOP", "Position (counts)"=0, "Velocity (0-1)"=0.0}) -> (w115:T26)
        }
        frame "Set Pose" {
          n148 = Unbundle By Name(w126) -> ("Pose Array"=w129:T1[], "Pose Index"=w128:i32)
          n149 = Index Array(array=w129, index=w128) -> (element=w116:T1)
          n150 = Unbundle By Name(w116) -> ("Lift"=w123:i32, "Extend"=w120:i32, "Wrist"=w119:i32)
          n151 = Bundle By Name(cluster=T6 {"Mode"=enum."Position", "Position (counts)"=0, "Velocity (0-1)"=0.0} ("Wrist CMD"), "Position (counts)"=w119) -> (w117:T6)
          n152 = Bundle By Name(cluster=T4 {"Mode"=enum."Position", "Position (counts)"=0, "Velocity (0-1)"=0.0} ("Extend CMD"), "Position (counts)"=w120) -> (w121:T4)
          n153 = Bundle By Name(cluster=T8 {"Mode"=enum."Position", "Position (counts)"=0, "Velocity (0-1)"=0.0} ("Sholder CMD"), "Position (counts)"=w123) -> (w124:T8)
          n154 = Bundle By Name(cluster=w126, "Current Pose"=w116, "Lift CMD"=w124, "Extend CMD"=w121, "Wrist CMD"=w117) -> (w127:T26)
        }
        frame "Config Pose Read File" {
        }
        frame "Build Pose List" {
          n155 = Unbundle By Name(w139) -> ("Current Pose"=w134:T1, "Config Data.Pose List"=w136:T11[], "CMD.Pose Target"=w141:T3, "CMD.Position Target"=w135:T1)
          n156 = call "Build Pose Target Array.vi"("Current Pose"=w134, "Pose Position Target"=w135, "Pose Name Target"=w141, "Pose Config"=w136) -> ("Valid Value Out"=w133:bool, "Pose Targets Out"=w137:T1[])  [unwired: 6 in]
          n157 = Bundle By Name(cluster=w139, "Pose Index"=0, "Pose Array"=w137, "Valid Pose Target"=w133, "MotionMaster_Output.Motion complete"=FALSE, "MotionMaster_Output.Timed Out"=FALSE) -> (w140:T26)
        }
        frame "Config SW File Read" {
          n158 = Unbundle By Name(w146) -> ("Team Files Folder"=w144:path, "Config Data"=w142:T10)
          n159 = call "RWA_File Config.vim"("Read(f) Write(t)"=FALSE, "Target Folder Folder"=w144, "Any Config"=w142) -> ("Any Config Out"=w145:T10)  [unwired: 4 in, 4 out]
          n160 = Bundle By Name(cluster=w146, "Config Data"=w145) -> (w147:T26)
        }
        frame "Config SW File Save" {
          n161 = Unbundle By Name(w152) -> ("Team Files Folder"=w150:path, "Config Data"=w148:T10)
          n162 = call "RWA_File Config.vim"("Read(f) Write(t)"=TRUE, "Target Folder Folder"=w150, "Any Config"=w148) -> ("Any Config Out"=w151:T10)  [unwired: 4 in, 4 out]
          n163 = Bundle By Name(cluster=w152, "Config Data"=w151) -> (w153:T26)
        }
        frame "Config From FP" {
          n164 = Unbundle By Name(w162) -> ("Current Time"=w163:timestamp)
          n165 = Unbundle By Name(w162) -> ("Config Data"=w161:T10, "Config Data.MotionMaster Ver"=w156:u64)
          n166 = Not Equal?(x="Config Data", y=w161) -> (x != y?=w158:bool)
          n167 = call "Date Stamp.vi"("Time"=w163) -> ("U64 Out"=w157:u64)  [unwired: 5 in, 1 out]
          n168 = Select(t=w157, s=w158, f=w156) -> (s? t:f=w155:u64)
          n169 = Bundle By Name(cluster="Config Data", "MotionMaster Ver"=w155) -> (w159:T10)
          n170 = Bundle By Name(cluster=w162, "Config Data"=w159, "Update Display"=TRUE) -> (w164:T26)
        }
      }
    }
    n171 = Unbundle By Name(w43) -> ("CMD.ENABLE"=w71:bool, "Previous CMD.ENABLE"=w68:bool)
    "CMD.ENABLE" <- w71
    n172 = Unbundle By Name(w43) -> ("CMD"=→"CMD":T12, "Current Time"=→"Current Time":timestamp, "Lift HW.Encoder.Position"=→"Lift Position":i32, "Lift SW.At Positon"=→"Lift @ Positon":bool, "Extend HW.FX Encoder.Position"=→"Extend Position":i32, "Extend SW.exAt Positon"=→"Extend @ Positon":bool, "Wrist HW.Encoder.Position"=→"Wrist Position":i32, "Wrist SW.Wr At Positon"=→"Wrist @Positon":bool)
    n173 = Unbundle By Name(w43) -> ("MotionMaster_Output"=w44:T2)
    "MotionMaster_Output" <- w44
    n174 = Unbundle By Name(w43) -> ("Pose Array"=→"Pose Targets":T1[], "Pose Index"=→"Pose Index":i32)
    n175 = Unbundle By Name(w43) -> ("Config Data"=w53:T10, "Update Display"=w54:bool)
    n176 = case shown="True" w71 {
      tunnel: w43 -> [_ w100]
      tunnel: w68 -> [w96 _]
      frame False {
        # "Disabled"
        n177 = case shown="True" w96 {
          frame False {
          }
          frame True {
            # "Falling Edge"
            n178 = global write "Global_CMD_ACT_Data In.vi" "CMD_ACT_Wrist Data"(T6 {"Mode"=enum."STOP", "Position (counts)"=0, "Velocity (0-1)"=0.0} ("CMD_Wrist_Template_Data")) -> ()
            n179 = global write "Global_CMD_ACT_Data In.vi" "CMD_ACT_Extend_Data"(T4 {"Mode"=enum."STOP", "Position (counts)"=0, "Velocity (0-1)"=0.0} ("CMD_ExtendTemplate_Data")) -> ()
            n180 = global write "Global_CMD_ACT_Data In.vi" "CMD_ACT_Lift_Data"(T8 {"Mode"=enum."STOP", "Position (counts)"=0, "Velocity (0-1)"=0.0} ("CMD_ACT_Sholder_Data")) -> ()
          }
        }
      }
      frame True {
        n181 = Unbundle By Name(w100) -> ("Lift CMD"=w102:T8, "Extend CMD"=w103:T4, "Wrist CMD"=w101:T6)
        "Lift CMD" <- w102
        "Wrist CMD" <- w101
        "Extend CMD" <- w103
        n182 = global write "Global_CMD_ACT_Data In.vi" "CMD_ACT_Lift_Data"(w102) -> ()
        n183 = global write "Global_CMD_ACT_Data In.vi" "CMD_ACT_Extend_Data"(w103) -> ()
        n184 = global write "Global_CMD_ACT_Data In.vi" "CMD_ACT_Wrist Data"(w101) -> ()
      }
    }
    n185 = case shown="True" w54 {
      tunnel: w53 -> [_ w95]
      frame False {
      }
      frame True {
        n186 = local write "Config Data"(w95) -> ()
      }
    }
    n187 = Unbundle By Name(w43) -> ("Cycle Time(S)"=w78:dbl)
    "Cycle Time (S)" <- w78
    n188 = global write "Global_CMD_Data Out.vi" "SubCMD_MotionMaster_Output"(w44) -> ()
    n189 = global write "Global_CMD_Data Out.vi" "SubCMD_MotionMaster_CycleTime(S)"(w78) -> ()
    n190 = Bundle By Name(cluster=w43, "Update Display"=FALSE) -> (w46:T26)
  }
  n191 = flat-sequence {
    frame #0 {
      (unwired) ENUM_CMD_State."Startup" ("State")
      (unwired) ENUM_CMD_Action."Set Pose" ("Action")
      # "State LIST"
      # "Action LIST"
    }
  }
